vi "Is Window Being Shown - Get.vi"() -> (0 "Is Error Window Currently Being Shown?":bool)   [LabVIEW 2023, in "Error Manager.lvlib" / "Error Display Window.lvclass"]
uses:
  Error Display Window.lvclass
  Is Window Being Shown (class variable).vi
  Error Display Window.lvclass/Error Display Window.ctl
panel:
  # "Development\ncontrols/indicators useful for development and testing, but which are not outputs of the VI"
  # "Input\nInputs to the VI"
  # "Output\nOutputs of the VI"
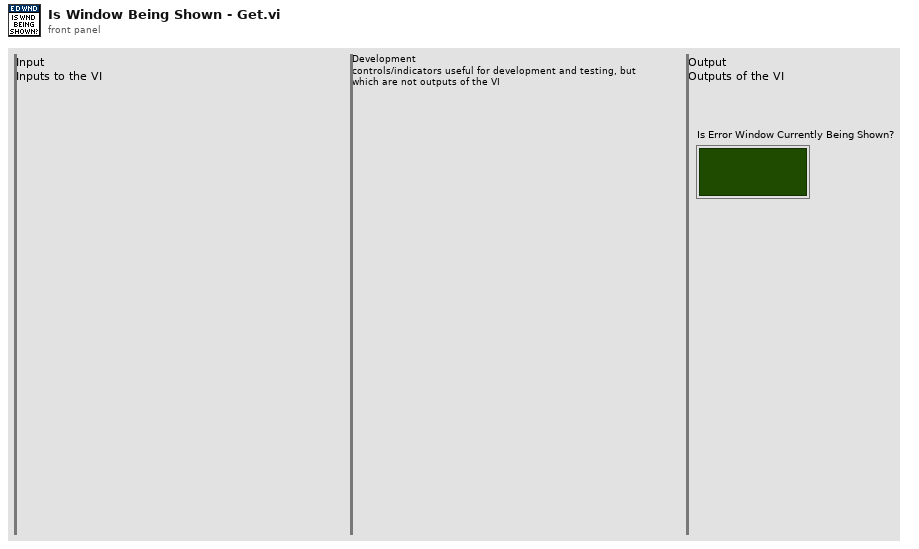
[diagram p1: front panel]
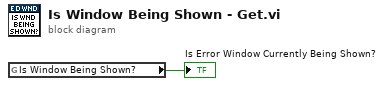
[diagram p0: block diagram]
diagram:
  n1 = global read "Is Window Being Shown (class variable).vi" "Is Window Being Shown?"() -> (→"Is Error Window Currently Being Shown?":bool)
